vi "小时数据主动发送(子VI).vi"   [LabVIEW 2016]
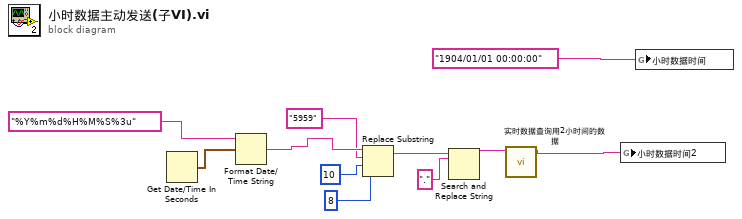
[diagram p0: block diagram]
diagram:
  n1 = Get Date/Time In Seconds() -> (seconds since 1Jan1904=w9:timestamp)
  n2 = Format Date/Time String(time format string (%c)="%Y%m%d%H%M%S%3u" ("时间格式字符串(%c)"), seconds (now)=w9) -> (date/time string=w11:string)  [unwired: 1 in]
  n3 = Replace Substring(2:8 ("长度（子字符串长度）"), 3:10 ("偏移量(0)"), 4:"5959" ("子字符串(\"\")"), 5:w11) -> (1:w3:string)  [unwired: 1 out]
  n4 = Search and Replace String(input string=w3, search string="." ("搜索字符串")) -> (result string=w2:string)  [unwired: 6 in, 3 out]
  n5 = call "实时数据查询用2小时间的数据.vi"("字符串"=w2) -> ("连接的字符串"=w1:string)  [unwired: 10 in]
  n6 = global write "全局 时间2.vi" "小时数据时间2"(w1) -> ()
  n7 = global write "全局 时间.vi" "小时数据时间"("1904/01/01 00:00:00") -> ()
